vi "Get Report Type.vi"(4 "error in (no error)":errorcluster, 7 "report in":T1) -> (0 "error out":errorcluster, 2 "output element":enum16{"Standard Report", "HTML"}(ring), 3 "report out":T1)   [LabVIEW 2017]
doc: "Determines whether the report is printed or HTML-based."
uses:
  <vilib>/Utility/NIReport.llb/Generate Report Object Reference.ctl
  <vilib>/Utility/NIReport.llb/NI_report.lvclass
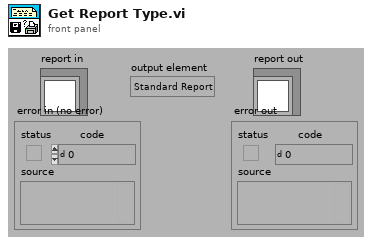
[diagram p1: front panel]
types:
  T1 = typedef "Generate Report Object Reference.ctl" = refnum<class "NI_report.lvclass">
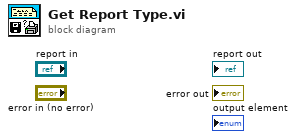
[diagram p0: block diagram]
diagram:
